vi "External Code (DLL) Execution.vi"() -> ()   [LabVIEW 2023]
doc: "This VI allows you to browse examples of external code (C and C++) data types and how they interface with LabVIEW. Each data type has an example VI that demonstrates the use of the Call Library Function Node. To open the example VI for a particular data type, select that data type from the list on the left and then press the \"Open Example VI for Current Data Type\" button. The function prototype, the function's source code, and any specific details about this example will appear in the External Code Information cluster."
panel:
  in  "Data Type Information":T1(array[cluster])=[{"Type"="BOOL", "LabVIEW Data Type"="I32", "Function Prototype"="void WinBOOL(BOOL input, BOOL *output);", "Base Filename"="WinBOOL", "Caution"="", "Summary"="This function inverts the value of input and returns it in output.\n\nNOTE: LPBOOL and PBOOL are equivalent to the BOOL* data type."}, {"Type"="BOOLEAN", "LabVIEW Data Type"="U8", "Function Prototype"="void WinBOOLEAN(BOOLEAN input, BOOLEAN *pinput, PBOOLEAN output);", "Base Filename"="WinBOOLEAN", "Caution"="If using Adapt to Type to wire booleans directly to and from the Call Library Function, note that all inputs will be passed by reference, not by value.", "Summary"="This function ANDs the input values input and pinput and returns the inverse of the result in output.\n\nNOTE: PBOOLEAN is equivalent to the BOOLEAN* data type."}, {"Type"="BYTE", "LabVIEW Data Type"="U8", "Function Prototype"="void WinBYTE(BYTE input, BYTE *output);", "Base Filename"="WinBYTE", "Caution"="", "Summary"="This function ANDs input with 0xAA and returns the result in output.\n\nNOTE: LPBYTE and PBYTE are equivalent to BYTE* data type."}, {"Type"="CHAR", "LabVIEW Data Type"="String", "Function Prototype"="void WinCHAR(CHAR *input, PCHAR output);", "Base Filename"="WinCHAR", "Caution"="This example is for character arrays, better known as strings. If you need to pass just a byte, use an U8 numeric value from LabVIEW or see the BYTE data type example.\n\nWhen returning a new character string from a DLL, you must allocate memory for the string in LabVIEW. The easiest way to do this is to input a string of a known length into the Call Library Function node that is at least as large as the expected resulting string being returned from the DLL. See the VI for one way to do this.", "Summary"="This function reverses the input string and places it in output.\n\nNOTE: PCHAR, LPCHAR, and PSTR are equivalent to the CHAR* data type. LPCSTR and PCSTR are pointers to constant strings and are equivalent to CONST CHAR* data type."}, {"Type"="COLORREF", "LabVIEW Data Type"="U32 with conversion", "Function Prototype"="void WinCOLORREF(COLORREF input, COLORREF *output);", "Base Filename"="WinCOLORREF", "Caution"="LabVIEW represents colors in a 0xRRGGBB format. Windows COLORREF data type is represented ar 0xBBGGRR. In the example VI, byte swapping is done so that the data in the DLL call is in the proper format. The resultant color is then byte swapped back to the LabVIEW format.", "Summary"="If input is black, then output will be blue. Otherwise, output will be green.\n\nNOTE: LPCOLORREF is equivalent to the COLORREF* data type."}, {"Type"="DWORD", "LabVIEW Data Type"="U32", "Function Prototype"="void WinDWORD(DWORD input, DWORD *output);", "Base Filename"="WinDWORD", "Caution"="", "Summary"="This function squares the value of input and returns the value in output.\n\nNOTE: PDWORD and LPDWORD are equivalent to the DWORD* data type. DWORD32 is equivalent to DWORD on 32-bit Windows operating systems."}, {"Type"="FLOAT", "LabVIEW Data Type"="SGL", "Function Prototype"="void WinFLOAT(FLOAT input, FLOAT *output);", "Base Filename"="WinFLOAT", "Caution"="This is for the Windows FLOAT type. This is equivalent to the ANSI float type, not the double type.", "Summary"="This function squares the value of input and returns the value in output.\n\nNOTE: PFLOAT is equivalent to the FLOAT* data type."}, {"Type"="HWND", "LabVIEW Data Type"="U32", "Function Prototype"="void WinHWND(char *name, HWND *output);", "Base Filename"="WinHWND", "Caution"="", "Summary"="This function flashes the example VI's title bar 5 times. The HWND for the example VI is returned in output."}, {"Type"="INT", "LabVIEW Data Type"="I32", "Function Prototype"="void WinINT(int input, int *output);", "Base Filename"="WinINT", "Caution"="", "Summary"="This function squares the value of input and returns the value in output.\n\nNOTE: PINT and LPINT are equivalent to the INT* data type. INT32 is equivalent to the INT data type. "}, {"Type"="LONG", "LabVIEW Data Type"="I32", "Function Prototype"="void WinLONG(LONG input, LONG *output);", "Base Filename"="WinLONG", "Caution"="", "Summary"="This function squares the value of input and returns the value in output.\n\nNOTE: PLONG and LPLONG are equivalent to the LONG* data type. LONG32 and LPARAM are equivalent to the LONG data type. "}, {"Type"="SHORT", "LabVIEW Data Type"="I16", "Function Prototype"="void WinSHORT(SHORT input, SHORT *output);", "Base Filename"="WinSHORT", "Caution"="", "Summary"="This function doubles the value of input and returns the value in output.\n\nNOTE: PSHORT is equivalent to the SHORT* data type."}, {"Type"="SIZE_T", "LabVIEW Data Type"="U32", "Function Prototype"="void WinSIZE_T(SIZE_T input, SIZE_T *output);", "Base Filename"="WinSIZE_T", "Caution"="", "Summary"="This function squares the value of input and returns the value in output."}, {"Type"="SSIZE_T", "LabVIEW Data Type"="I32", "Function Prototype"="void WinSSIZE_T(SSIZE_T input, SSIZE_T *output);", "Base Filename"="WinSSIZE_T", "Caution"="", "Summary"="This function squares the value of input and returns the value in output."}, {"Type"="UCHAR", "LabVIEW Data Type"="String", "Function Prototype"="void WinUCHAR(UCHAR *input, PUCHAR output);", "Base Filename"="WinUCHAR", "Caution"="This example is for character arrays, better known as strings. If you need to pass just a byte, use an U8 numeric value from LabVIEW or see the BYTE data type example.\n\nWhen returning a new character string from a DLL, you must allocate memory for the string in LabVIEW. The easiest way to do this is to input a string of a known length into the Call Library Function node that is at least as large as the expected resulting string being returned from the DLL. See the VI for one way to do this.", "Summary"="This function reverses the input string and places it in output.\n\nNOTE: PUCHAR is equivalent to the UCHAR* data type."}, {"Type"="UINT", "LabVIEW Data Type"="U32", "Function Prototype"="void WinUINT(UINT input, UINT *output);", "Base Filename"="WinUINT", "Caution"="", "Summary"="This function squares the value of input and returns the value in output.\n\nNOTE: PUINT is equivalent to the UINT* data type. UINT32 is equivalent to the INT data type. "}, {"Type"="ULONG", "LabVIEW Data Type"="U32", "Function Prototype"="void WinULONG(ULONG input, ULONG *output);", "Base Filename"="WinULONG", "Caution"="", "Summary"="This function squares the value of input and returns the value in output.\n\nNOTE: PULONG is equivalent to the ULONG* data type. ULONG32 and WPARAM are equivalent to the ULONG data type. "}, {"Type"="USHORT", "LabVIEW Data Type"="U16", "Function Prototype"="void WinUSHORT(USHORT input, USHORT *output);", "Base Filename"="WinUSHORT", "Caution"="", "Summary"="This function doubles the value of input and returns the value in output.\n\nNOTE: PUSHORT is equivalent to the USHORT* data type."}, {"Type"="WORD", "LabVIEW Data Type"="U16", "Function Prototype"="void WinWORD(WORD input, WORD *output);", "Base Filename"="WinWORD", "Caution"="", "Summary"="This function doubles the value of input and returns the value in output.\n\nNOTE: PWORD and LPWORD are equivalent to the WORD* data type."}, {"Type"="char", "LabVIEW Data Type"="String", "Function Prototype"="void ANSIchar(char *input, char *output);", "Base Filename"="ANSIchar", "Caution"="This example is for character arrays, better known as strings. If you need to pass just a byte, use an I8 numeric value from LabVIEW or see the BYTE data type example for Windows Data Types.\n\nWhen returning a new character string from a DLL, you must allocate memory for the string in LabVIEW. The easiest way to do this is to input a string of a known length into the Call Library Function node that is at least as large as the expected resulting string being returned from the DLL. See the VI for one way to do this.", "Summary"="This function reverses the input string and places it in output."}, {"Type"="double", "LabVIEW Data Type"="DBL", "Function Prototype"="void ANSIdouble(double input, double *output);", "Base Filename"="ANSIdouble", "Caution"="", "Summary"="This function squares the value of input and returns the value in output."}, {"Type"="float", "LabVIEW Data Type"="SGL", "Function Prototype"="void ANSIfloat(float input, float *output);", "Base Filename"="ANSIfloat", "Caution"="", "Summary"="This function squares the value of input and returns the value in output."}, {"Type"="int", "LabVIEW Data Type"="I32", "Function Prototype"="void ANSIint(int input, int *output);", "Base Filename"="ANSIint", "Caution"="", "Summary"="This function squares the value of input and returns the value in output."}, {"Type"="long", "LabVIEW Data Type"="I32", "Function Prototype"="void ANSIlong(long input, long *output);", "Base Filename"="ANSIlong", "Caution"="", "Summary"="This function squares the value of input and returns the value in output."}, {"Type"="short", "LabVIEW Data Type"="I16", "Function Prototype"="void ANSIshort(short input, short *output", "Base Filename"="ANSIshort", "Caution"="", "Summary"="This function doubles the value of input and returns the value in output."}, {"Type"="unsigned char", "LabVIEW Data Type"="String", "Function Prototype"="void ANSIunsignedchar(insigned char *input, unsigned char *output);", "Base Filename"="ANSIunsignedchar", "Caution"="This example is for character arrays, better known as strings. If you need to pass just a byte, use an U8 numeric value from LabVIEW or see the BYTE data type example for Windows Data Types.\n\nWhen returning a new character string from a DLL, you must allocate memory for the string in LabVIEW. The easiest way to do this is to input a string of a known length into the Call Library Function node that is at least as large as the expected resulting string being returned from the DLL. See the VI for one way to do this.", "Summary"="This function reverses the input string and places it in output."}, {"Type"="unsigned int", "LabVIEW Data Type"="U32", "Function Prototype"="void ANSIunsignedint(unsigned int input, unsigned int *output);", "Base Filename"="ANSIunsignedint", "Caution"="", "Summary"="This function squares the value of input and returns the value in output."}, {"Type"="unsigned long", "LabVIEW Data Type"="U32", "Function Prototype"="void ANSIunsignedlong(unsigned long input, unsigned long *output);", "Base Filename"="ANSIunsignedlong", "Caution"="", "Summary"="This function squares the value of input and returns the value in output."}, {"Type"="unsigned short", "LabVIEW Data Type"="U16", "Function Prototype"="void ANSIunsignedshort(unsigned short input, unsigned short *output);", "Base Filename"="ANSIunsignedshort", "Caution"="", "Summary"="This function doubles the value of input and returns the value in output."}, {"Type"="cmplx64", "LabVIEW Data Type"="CSG", "Function Prototype"="void LVcmplx64(cmplx64 input, cmplx64 *output);", "Base Filename"="LVcmplx64", "Caution"="", "Summary"="This function squares the value of input and returns the value in output."}, {"Type"="cmplx128", "LabVIEW Data Type"="CDB", "Function Prototype"="void LVcmplx128(cmplx128 input, cmplx128 *output);", "Base Filename"="LVcmplx128", "Caution"="", "Summary"="This function squares the value of input and returns the value in output."}, {"Type"="cmplxExt", "LabVIEW Data Type"="CXT", "Function Prototype"="void LVcmplxExt(cmplxEXT input, cmplxExt *output);", "Base Filename"="LVcmplx128", "Caution"="", "Summary"="This function doubles the value of input and returns the value in output."}, {"Type"="CStr", "LabVIEW Data Type"="String", "Function Prototype"="void LVCStr(CStr input, CStr output);", "Base Filename"="LVCStr", "Caution"="", "Summary"="This function reverses the input string and places it in output.\n\nNOTE: CStr is equivalent to the unsigned char* data type."}, {"Type"="float32", "LabVIEW Data Type"="SGL", "Function Prototype"="void LVfloat32(float32 input, float32 *output);", "Base Filename"="LVfloat32", "Caution"="", "Summary"="This function squares the value of input and returns the value in output."}, {"Type"="float64", "LabVIEW Data Type"="DBL", "Function Prototype"="void LVfloat64(float64 input, float64 *output);", "Base Filename"="LVfloat64", "Caution"="", "Summary"="This function squares the value of input and returns the value in output."}, {"Type"="floatExt", "LabVIEW Data Type"="EXT", "Function Prototype"="void LVfloatExt(floatExt input, floatExt *output);", "Base Filename"="LVfloatExt", "Caution"="", "Summary"="This function doubles the value of input and returns the value in output."}, {"Type"="int8", "LabVIEW Data Type"="I8", "Function Prototype"="void LVint8(int8 input, int8 *output);", "Base Filename"="LVint8", "Caution"="", "Summary"="This function doubles the value of input and returns the value in output."}, {"Type"="int16", "LabVIEW Data Type"="I16", "Function Prototype"="void LVint16(int16 input, int16 *output);", "Base Filename"="LVint16", "Caution"="", "Summary"="This function doubles the value of input and returns the value in output."}, {"Type"="int32", "LabVIEW Data Type"="I32", "Function Prototype"="void LVint32(int32 input, int32 *output);", "Base Filename"="LVint32", "Caution"="", "Summary"="This function squares the value of input and returns the value in output."}, {"Type"="LStrHandle", "LabVIEW Data Type"="String", "Function Prototype"="void LVLStrHandle(LStrHandle input, LStrHandle output);", "Base Filename"="LVLStrHandle", "Caution"="The LStrHandle data type is composed of two parts:\n4 byte containing the length of the string\nArray of characters representing the string with no terminating character\n\nWhen returning a new character string from a DLL, you must allocate memory for the string in LabVIEW. The easiest way to do this is to input a string of a known length into the Call Library Function node that is at least as large as the expected resulting string being returned from the DLL. See the VI for one way to do this.", "Summary"="This function reverses the input string, concatenates it to the original string, and places it in output."}, {"Type"="LVBoolean", "LabVIEW Data Type"="Boolean", "Function Prototype"="void LVLVBoolean(LVBoolean input, LVBoolean *pinput, LVBoolean *output);", "Base Filename"="LVLVBoolean", "Caution"="If using Adapt to Type to wire booleans directly to and from the Call Library Function, note that all inputs will be passed by reference, not by value.", "Summary"="This function ANDs the input values input and pinput and returns the inverse of the result in output.\n"}, {"Type"="uInt8", "LabVIEW Data Type"="U8", "Function Prototype"="void LVuInt8(uInt8 input, uInt8 *output);", "Base Filename"="LVuInt8", "Caution"="", "Summary"="This function doubles the value of input and returns the value in output."}, {"Type"="uInt16", "LabVIEW Data Type"="U16", "Function Prototype"="void LVuInt16(uInt16 input, uInt16 *output);", "Base Filename"="LVuInt16", "Caution"="", "Summary"="This function doubles the value of input and returns the value in output."}, {"Type"="uInt32", "LabVIEW Data Type"="U32", "Function Prototype"="void LVuInt32(uInt32 input, uInt32 *output);", "Base Filename"="LVuInt32", "Caution"="", "Summary"="This function squares the value of input and returns the value in output."}, {"Type"="1-D Array", "LabVIEW Data Type"="1-D Array", "Function Prototype"="void ARRAYfloor1D(double *input, int input_length, int *output);", "Base Filename"="ARRAYfloor1D", "Caution"="When returning a new array from a DLL, you must allocate memory for the array in LabVIEW. The easiest way to do this is to input an array of a known length into the Call Library Function node that is at least as large as the expected resulting array being returned from the DLL. See the VI for one way to do this.\n\nIf the size of the returning array cannot be known before the Call Library Function node, then use of the memory management functions found in the \"Using External Code in LabVIEW\" manual is recommended. These functions would need to be used either in the original source code for the DLL or inside of a wrapper DLL that is called by LabVIEW. The wrapper DLL would then call the original DLL function in the original DLL.", "Summary"="This function gets the floor of the square of all element values in input and returns them in output. This VI demonstrates preallocating array memory for a separate, returned array.\n\nThis function uses the double and int data types. Any data type in LabVIEW can be used in a 1-D array in similar fashion."}, {"Type"="2-D Array", "LabVIEW Data Type"="2-D Array", "Function Prototype"="void ARRAY2D(double *array, int array_length_row, int array_length_col);", "Base Filename"="ARRAY2D", "Caution"="A 2-D array passed from LabVIEW as an array data pointer will be passed to the DLL as a 1-D array. Pointer arithmetic can be used to access this array as a 2-D array. See the VI for an example.\n\nWhen returning a new array from a DLL, you must allocate memory for the array in LabVIEW. The easiest way to do this is to input an array of a known length into the Call Library Function node that is at least as large as the expected resulting array being returned from the DLL. See the 1-D Array example for one way to do this.\n\nIf the size of the returning array cannot be known before the Call Library Function node, then use of the memory management functions found in the \"Using External Code in LabVIEW\" manual is recommended. These functions would need to be used either in the original source code for the DLL or inside of a wrapper DLL that is called by LabVIEW. The wrapper DLL would then call the original DLL function in the original DLL.", "Summary"="This function squares each value in the 2-D array.\n\nThis function uses the double data type. Any data type in LabVIEW can be used in a 2-D array in similar fashion.\n\nFor information on returning a new array to LabVIEW, see the 1-D Array example."}, {"Type"="3-D Array", "LabVIEW Data Type"="3-D Array", "Function Prototype"="void ARRAY3D(double *array, int array_length_page, int array_length_row, int array_length_col);", "Base Filename"="ARRAY3D", "Caution"="A 3-D array passed from LabVIEW as an array data pointer will be passed to the DLL as a 1-D array. Pointer arithmetic can be used to access this array as a 3-D array. See the VI for an example.\n\nWhen returning a new array from a DLL, you must allocate memory for the array in LabVIEW. The easiest way to do this is to input an array of a known length into the Call Library Function node that is at least as large as the expected resulting array being returned from the DLL. See the 1-D Array example for one way to do this.\n\nIf the size of the returning array cannot be known before the Call Library Function node, then use of the memory management functions found in the \"Using External Code in LabVIEW\" manual is recommended. These functions would need to be used either in the original source code for the DLL or inside of a wrapper DLL that is called by LabVIEW. The wrapper DLL would then call the original DLL function in the original DLL.", "Summary"="This function sums each element in pages 0 through n-2 of an n page sized 3-D array and places the values in the corresponding element on page n-1. It is assumed that page n-1 is already allocated in the input array.\n\nThis function uses the double data type. Any data type in LabVIEW can be used in a 3-D array in similar fashion.\n\nFor information on returning a new array to LabVIEW, see the 1-D Array example."}, {"Type"="1-D Array Handle", "LabVIEW Data Type"="1-D Array", "Function Prototype"="void ARRAY1DHandle(TD1Hdl input, TD2Hdl output);", "Base Filename"="ARRAY1DHandle", "Caution"="When returning a new array from a DLL, you must allocate memory for the array in LabVIEW. The easiest way to do this is to input an array of a known length into the Call Library Function node that is at least as large as the expected resulting array being returned from the DLL. See the VI for one way to do this.\n\nIf the size of the returning array cannot be known before the Call Library Function node, then use of the memory management functions found in the \"Using External Code in LabVIEW\" manual is recommended. These functions would need to be used either in the original source code for the DLL or inside of a wrapper DLL that is called by LabVIEW. The wrapper DLL would then call the original DLL function in the original DLL.", "Summary"="This function gets the floor of the square of all element values in input and returns them in output. This VI demonstrates preallocating array memory for a separate, returned array.\n\nThis function uses the double and int data types. Any data type in LabVIEW can be used in a 1-D array in similar fashion.\n\nWhen using array handle types in LabVIEW, it is best to have LabVIEW create the skeleton .c file for you by right-clicking on the Call Library Function node and selecting Create .c File.... This is how the type descriptor structures were created for this example."}, {"Type"="2-D Array Handle", "LabVIEW Data Type"="2-D Array", "Function Prototype"="void ARRAY2DHandle(TD1Hdl array);", "Base Filename"="ARRAY2DHandle", "Caution"="When returning a new array from a DLL, you must allocate memory for the array in LabVIEW. The easiest way to do this is to input an array of a known length into the Call Library Function node that is at least as large as the expected resulting array being returned from the DLL. See the 1-D Array Handle example for one way to do this.\n\nIf the size of the returning array cannot be known before the Call Library Function node, then use of the memory management functions found in the \"Using External Code in LabVIEW\" manual is recommended. These functions would need to be used either in the original source code for the DLL or inside of a wrapper DLL that is called by LabVIEW. The wrapper DLL would then call the original DLL function in the original DLL.", "Summary"="This function squares each value in the 2-D array.\n\nThis function uses the double data type. Any data type in LabVIEW can be used in a 2-D array in similar fashion.\n\nFor information on returning a new array to LabVIEW, see the 1-D Array Handle example.\n\nWhen using array handle types in LabVIEW, it is best to have LabVIEW create the skeleton .c file for you by right-clicking on the Call Library Function node and selecting Create .c File.... This is how the type descriptor structures were created for this example."}, {"Type"="3-D Array Handle", "LabVIEW Data Type"="3-D Array", "Function Prototype"="void ARRAY3D(TD1Hdl array);", "Base Filename"="ARRAY3DHandle", "Caution"="When returning a new array from a DLL, you must allocate memory for the array in LabVIEW. The easiest way to do this is to input an array of a known length into the Call Library Function node that is at least as large as the expected resulting array being returned from the DLL. See the 1-D Array Handle example for one way to do this.\n\nIf the size of the returning array cannot be known before the Call Library Function node, then use of the memory management functions found in the \"Using External Code in LabVIEW\" manual is recommended. These functions would need to be used either in the original source code for the DLL or inside of a wrapper DLL that is called by LabVIEW. The wrapper DLL would then call the original DLL function in the original DLL.", "Summary"="This function sums each element in pages 0 through n-2 of an n page sized 3-D array and places the values in the corresponding element on page n-1. It is assumed that page n-1 is already allocated in the input array.\n\nThis function uses the double data type. Any data type in LabVIEW can be used in a 3-D array in similar fashion.\n\nFor information on returning a new array to LabVIEW, see the 1-D Array Handle example.\n\nWhen using array handle types in LabVIEW, it is best to have LabVIEW create the skeleton .c file for you by right-clicking on the Call Library Function node and selecting Create .c File.... This is how the type descriptor structures were created for this example."}, {"Type"="Simple Cluster", "LabVIEW Data Type"="Cluster", "Function Prototype"="void CLUSTERSimple(TD1 *input, TD1 *output);", "Base Filename"="CLUSTERSimple", "Caution"="When returning a new cluster from a DLL, you must allocate memory for the cluster in LabVIEW. The easiest way to do this is to input a cluster of a known type into the Call Library Function node that is the same as the expected resulting cluster being returned from the DLL. If you are returning the result to a control, then the control's memory is sufficient for this purpose when the cluster does not contain arrays or strings.\n\nTo dynamically create a cluster inside of the DLL, using the memory management functions found in the \"Using External Code in LabVIEW\" manual is recommended. These functions would need to be used either in the original source code for the DLL or inside of a wrapper DLL that is called by LabVIEW. The wrapper DLL would then call the original DLL function in the original DLL.", "Summary"="This function takes a cluster that contains a DBL, I32, and Boolean (in that order) as input. It squares the value of the DBL, halves the value of the I32, and NOTs the Boolean. The result is returned in output.\n\nThis function demonstrates how to call a structure that contains only simple data types. These would include floating points, integers, complex values, and booleans. Also, a single character is included in this list, but a string is not. Arrays are also not covered. \n\nFor structures that contain an inline array(s) and/or string(s) see the Simple Cluster String & Array example. For structures that contain pointers to array(s) and/or string(s) see the Complex example."}, {"Type"="Simple Cluster\nString & Array", "LabVIEW Data Type"="Cluster", "Function Prototype"="void CLUSTERSimpleS_A(TD1 *input, TD1 *output);", "Base Filename"="CLUSTERSimpleS_A", "Caution"="When returning a new cluster from a DLL, you must allocate memory for the cluster in LabVIEW. The easiest way to do this is to input a cluster of a known type into the Call Library Function node that is the same as the expected resulting cluster being returned from the DLL. If you are returning the result to a control, then the control's memory is sufficient for this purpose when the cluster does not contain arrays or strings.\n\nIf the cluster contains arrays or stings, then the easiest method is to create either a block diagram contstant of the cluster type. Each array should have enough elements allocated (not grayed out) to accommodate the returned array. In the same way, each string should have enough NULL characters in it to accommodate the returned string. See the VI for one way to do this.\n\nTo dynamically create a cluster inside of the DLL, using the memory management functions found in the \"Using External Code in LabVIEW\" manual is recommended. These functions would need to be used either in the original source code for the DLL or inside of a wrapper DLL that is called by LabVIEW. The wrapper DLL would then call the original DLL function in the original DLL.", "Summary"="This function takes a cluster that contains a DBL, string, and array of I32 (in that order)\nas input. It squares the value of the DBL, reverses the string, and doubles the value of each element in the array. The result is returned in output.\n\nThis function uses embedded, inline clusters of simple data types to imitate the contiguous memory used by an inline srting and/or array. Another method is to use a wrapper function and separate the LabVIEW data types in external code and pass a new structure to the original function. To see this example, see the Simple Cluster String & Array with Wrapper example.\n\nFor structures that do not contain an inline array(s) and/or string(s) see the Simple Cluster example. For structures that contain pointers to array(s) and/or string(s) see the Complex Cluster example."}, {"Type"="Simple Cluster\nString & Array\nwith Wrapper", "LabVIEW Data Type"="Cluster", "Function Prototype"="void CLUSTERSimpleS_AWrap(TD2 *input, TD2 *output);", "Base Filename"="CLUSTERSimpleS_AWrap", "Caution"="When returning a new cluster from a DLL, you must allocate memory for the cluster in LabVIEW. The easiest way to do this is to input a cluster of a known type into the Call Library Function node that is the same as the expected resulting cluster being returned from the DLL. If you are returning the result to a control, then the control's memory is sufficient for this purpose when the cluster does not contain arrays or strings.\n\nIf the cluster contains arrays or stings, then the easiest method is to create either a block diagram contstant of the cluster type. Each array should have enough elements allocated (not grayed out) to accommodate the returned array. In the same way, each string should have enough NULL characters in it to accommodate the returned string. See the Simple Cluster String & Array example for one way to do this.\n\nTo dynamically create a cluster inside of the DLL, using the memory management functions found in the \"Using External Code in LabVIEW\" manual is recommended. These functions would need to be used either in the original source code for the DLL or inside of a wrapper DLL that is called by LabVIEW. The wrapper DLL would then call the original DLL function in the original DLL.", "Summary"="This function takes a cluster that contains a DBL, string, and array of I32 (in that order) as input. It squares the value of the DBL, reverses the string, and doubles the value of each element in the array. The result is returned in output.\n\nThis function uses a wrapper function to separate the LabVIEW data types in external code and pass a new structure to the original function. Another method is to use embedded, inline clusters of simple data types to imitate the contiguous memory used by an inline srting and/or array. To see this example, see the Simple Cluster String & Array example.\n\nFor structures that do not contain an inline array(s) and/or string(s) see the Simple Cluster example. For structures that contain pointers to array(s) and/or string(s) see the Complex Cluster example."}, {"Type"="Complex Cluster", "LabVIEW Data Type"="Cluster", "Function Prototype"="void CLUSTERComplex(TD2 *input, TD2 *output);", "Base Filename"="CLUSTERComplex", "Caution"="When returning a new cluster from a DLL, you must allocate memory for the cluster in LabVIEW. The easiest way to do this is to input a cluster of a known type into the Call Library Function node that is the same as the expected resulting cluster being returned from the DLL. If you are returning the result to a control, then the control's memory is sufficient for this purpose when the cluster does not contain arrays or strings.\n\nIf the cluster contains arrays or stings, then the easiest method is to create either a block diagram contstant of the cluster type. Each array should have enough elements allocated (not grayed out) to accommodate the returned array. In the same way, each string should have enough NULL characters in it to accommodate the returned string. See the Simple Cluster String & Array example for one way to do this.\n\nTo dynamically create a cluster inside of the DLL, using the memory management functions found in the \"Using External Code in LabVIEW\" manual is recommended. These functions would need to be used either in the original source code for the DLL or inside of a wrapper DLL that is called by LabVIEW. The wrapper DLL would then call the original DLL function in the original DLL.", "Summary"="This function takes a cluster that contains a DBL, string, and array of I32 (in that order) as input (the string and array items are pointers to data outside of the structure). It squares the value of the DBL, reverses the input string and concatinates the reversed string to the original string, and doubles the value of each element in the array. The result is returned in output.\n\nThis function uses a wrapper function to separate the LabVIEW data types in external code and pass a new structure to the original function. This method must be used when the structure contains pointers to arrays and or strings.\n\nFor structures that do not contain an inline array(s) and/or string(s) see the Simple Cluster example. For structures that contain inline array(s) and/or string(s) see the Simple Cluster String & Array example."}, {"Type"="Cluster with\nnon-1-byte packing", "LabVIEW Data Type"="Cluster", "Function Prototype"="void CLUSTERBytePack#(TD# *input, TD# *output);", "Base Filename"="CLUSTERBytePack", "Caution"="Many Windows based DLLs have structures that are byte packed (#pragma pack(8)) at 8-byte intervals. LabVIEW expects the clusters it deals with to be packed at 1-byte intervals. This can cause issues ranging from wrong results to program crashes. If you call a DLL and have eliminated nearly every other possibility, check the byte packing of the structures. If they are packed at something other than 1-byte intervals, then use the VI as an example of a simple workaround.", "Summary"="This function takes a cluster that contains a DBL, Boolean, and I32 (in that order) as input. It squares the value of the DBL, halves the value of the I32, and NOTs the Boolean. The result is returned in output.\n\nThe 1-byte packed function allows a structure to have any data order because each data item will be placed directly after the previous item in memory. The 8-byte packed function has each data item packed on an 8-byte aligned value or the natural alignment of the data type, which ever is smaller. For instance, it the structure used in this example were ordered as DBL, I32, and Boolean, you would not see any difference in the results between the 8-byte or 1-byte function. In this instance, because the Boolean is before the I32, there is a 3-byte pad (because of natural alignment) in the 8-byte function. Since LabVIEW is expecting 1-byte packing, it stores the cluster to memory that way. When the DLL function reads the data, it is expecting an 8-byte packing order so the last value (I32) is incorrect."}]
  out "Summary":string
  out "Caution":string
  out "DLL Source Code":string
  out "Function Prototype":string
  in  "Stop":bool
  in  "Type List":i32(listbox)
  # "Overview: Demonstrates how to interface data types between external code (DLLs) and LabVIEW with the Call Library Function Node.\nRequirements: Windows\nInstructions:\n1. Run the VI.\n2. Single-click an item in the list to view information on a particular data type.\n3. Double-click an item in the list to open an example VI that demonstrates how to access that data type with a Call Library Function Node.\n4. Click Stop to stop the VI."
  # "See the Calling Shared Libraries topic in the LabVIEW Help for more information."
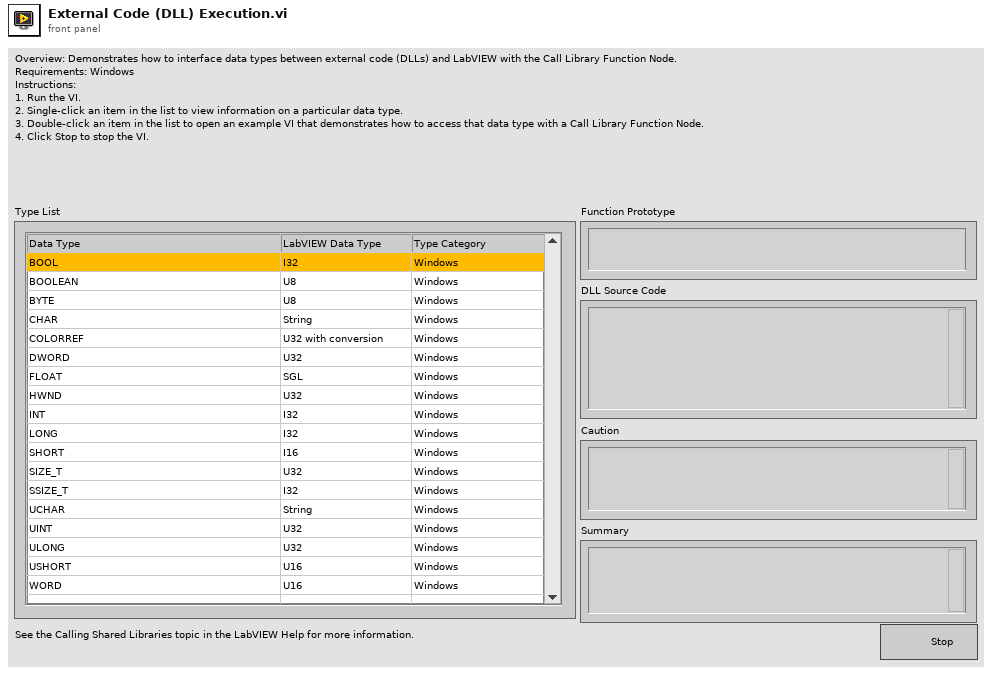
[diagram p1: front panel]
types:
  T1 = cluster{"Type":string, "LabVIEW Data Type":string, "Function Prototype":string, "Base Filename":string, "Caution":string, "Summary":string}[]
  T2 = cluster{"Type":string, "LabVIEW Data Type":string, "Function Prototype":string, "Base Filename":string, "Caution":string, "Summary":string}
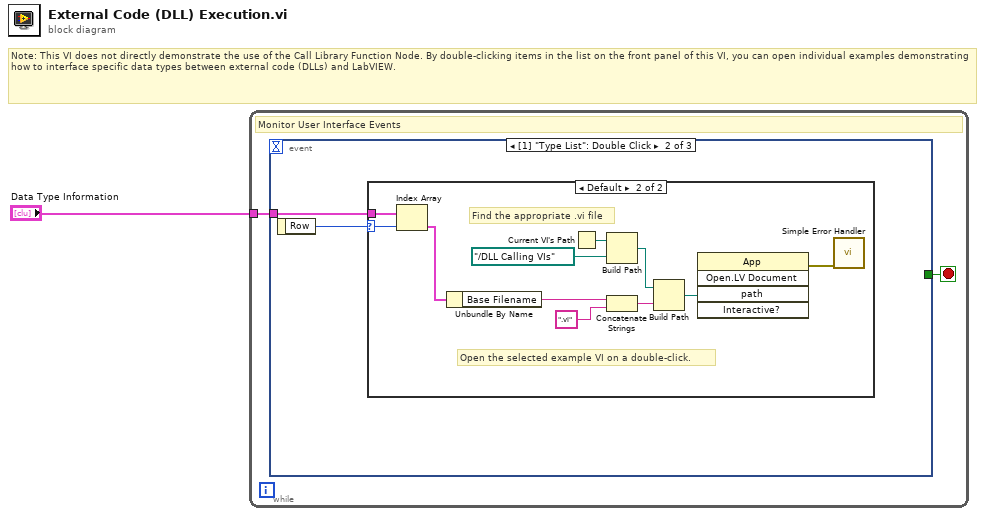
[diagram p0: block diagram]
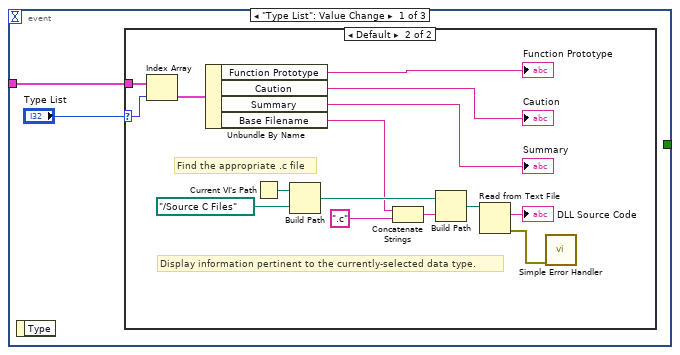
[diagram p2: hidden frame]
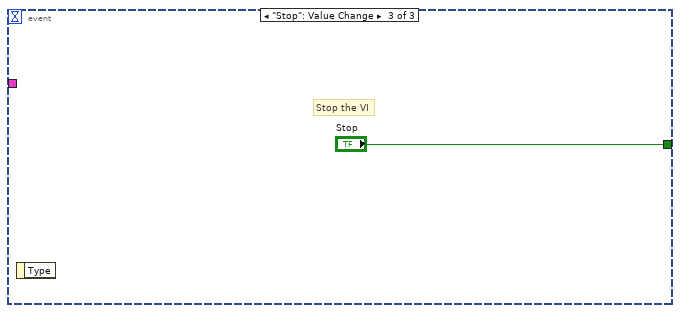
[diagram p5: hidden frame]
diagram:
  # "Note: This VI does not directly demonstrate the use of the Call Library Function Node. By double-clicking items in the list on the front panel of this VI, you can open individual examples demonstrating how to interface specific data types between external code (DLLs) and LabVIEW."
  n1 = while {
    tunnel: "Data Type Information" -> [w2]
    stop <- w3 stop-if-true
    # "Monitor User Interface Events"
    n2 = event shown="[1] \"Type List\": Double Click" {
      selector: _ -> [_ _ _]
      dyn-events: _ -> [_ _ _]
      timeout: _ -> [_ _ _]
      tunnel: [_ _ "Stop"] -> w3
      tunnel: w2 -> [w5 w22 _]
      event "Type List": Value Change {
        n3 = event-data() -> ()  [unwired: 1 in, 1 out]
        n4 = case shown="Default" "Type List" {
          selector: "Type List" -> [_ w6]
          tunnel: w5 -> [_ w16]
          frame ..-1 {
            # "Ignore value change if there is no selection in the listbox."
          }
          frame Default {
            # "Find the appropriate .c file"
            # "Display information pertinent to the currently-selected data type."
            n5 = Index Array(array=w16, index=w6) -> (element=w19:T2)
            n6 = Unbundle By Name(w19) -> ("Function Prototype"=→"Function Prototype":string, "Caution"=→"Caution":string, "Summary"=→"Summary":string, "Base Filename"=w8:string)
            n7 = Current VI's Path() -> (path=w10:path)
            n8 = Build Path(base path=w10, name or relative path=path "../Source C Files") -> (appended path=w20:path)
            n9 = Concatenate Strings(w8, ".c" ("string")) -> (w17:string)
            n10 = Build Path(base path=w20, name or relative path=w17) -> (appended path=w11:path)
            n11 = Read from Text File(file (use dialog)=w11) -> (text=→"DLL Source Code":string, error out=w7:errorcluster)  [unwired: 3 in, 2 out]
            n12 = call <vilib>:"Simple Error Handler.vi"("error in (no error)"=w7) -> ()  [unwired: 4 in, 5 out]
          }
        }
      }
      event "Type List": Double Click {
        n13 = event-data() -> ("Row"=w21:i32)  [unwired: 1 in]
        n14 = case shown="Default" w21 {
          selector: w21 -> [_ w23]
          tunnel: w22 -> [_ w27]
          frame ..-1 {
            # "Ignore double click if there is no selection in the listbox."
          }
          frame Default {
            # "Find the appropriate .vi file"
            # "Open the selected example VI on a double-click."
            n15 = Index Array(array=w27, index=w23) -> (element=w31:T2)
            n16 = Unbundle By Name(w31) -> ("Base Filename"=w33:string)
            n17 = Current VI's Path() -> (path=w26:path)
            n18 = Build Path(base path=w26, name or relative path=path "../DLL Calling VIs") -> (appended path=w32:path)
            n19 = Concatenate Strings(w33, ".vi" ("string")) -> (w29:string)
            n20 = Build Path(base path=w32, name or relative path=w29) -> (appended path=w28:path)
            n21 = invoke class="App" method="Open.LV Document"("path"=w28) -> (error out=w24:errorcluster)  [unwired: 4 in, 4 out]
            n22 = call <vilib>:"Simple Error Handler.vi"("error in (no error)"=w24) -> ()  [unwired: 4 in, 5 out]
          }
        }
      }
      event "Stop": Value Change {
        # "Stop the VI"
        n23 = event-data() -> ()  [unwired: 1 in, 1 out]
      }
    }
  }
